vi "Set Status Q.vi"(8 "error in (no error)":errorcluster, 10 "Status Q":refnum<class "MessageQ.lvclass">, 11 "Module in":refnum<class "Module.lvclass">) -> (0 "error out":errorcluster, 3 "Module out":refnum<class "Module.lvclass">)   [LabVIEW 2020, in "Volatus.lvlib" / "Module.lvclass"]
uses:
  Module.lvclass
  Module.lvclass/Module.ctl
  MessageQ/MessageQ.lvclass
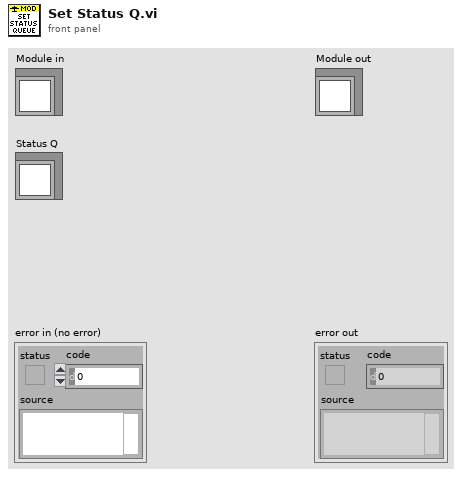
[diagram p1: front panel]
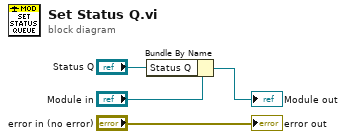
[diagram p0: block diagram]
diagram:
  n1 = Bundle By Name(cluster="Module in", "Status Q"="Status Q") -> (→"Module out":refnum<class "Module.lvclass">)
  "error out" <- "error in (no error)"
